vi "create queue client.vi"(8 "error in":errorcluster, 11 "conn string":string) -> (0 "error out":errorcluster, 3 "TCP client out":refnum<class "Queue client.lvclass">)   [LabVIEW 2015, in "Queue client.lvclass"]
uses:
  Queue client.lvclass
  client/connection client.lvclass/connection client.ctl
  client/connection client.lvclass
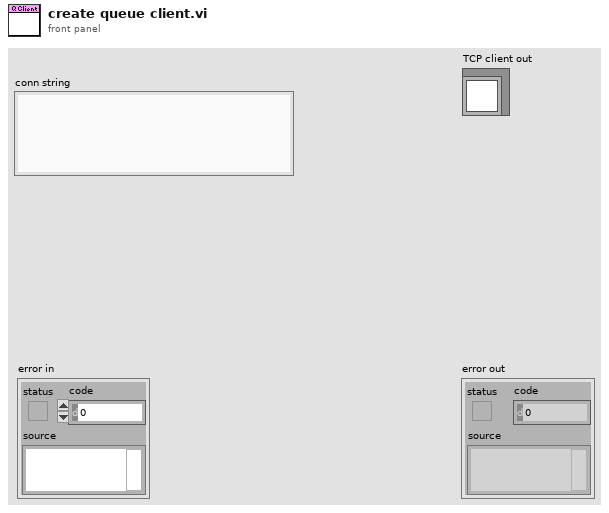
[diagram p1: front panel]
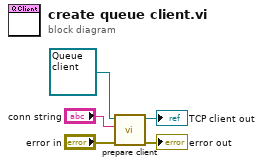
[diagram p0: block diagram]
diagram:
  n1 = call "prepare client.vi"("error in"="error in", "connection string"="conn string", "connection client in"=refnum<class "Queue client.lvclass"> refnum ("TCP client in")) -> ("error out"=→"error out":errorcluster, "connection client out"=→"TCP client out":refnum<class "Queue client.lvclass">)  [unwired: 7 in]
